vi "Pockels Cal-Reload file.vi"(8 "error in (no error)":errorcluster, 11 "Cal files listbox":refnum<vi>) -> (0 "error out":errorcluster, 3 "All data loaded":string[][](array[string]))   [LabVIEW 2020]
uses:
  Typedefs/Which path.ctl
  <userlib>/My Palettes.lib/Files & paths/Spreadsheet/Read From Spreadsheet File (string)-Mod.vi
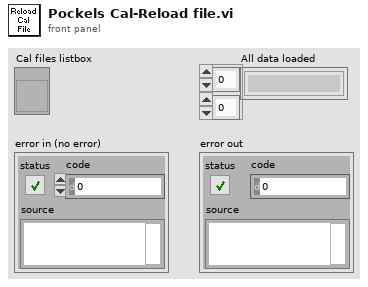
[diagram p1: front panel]
types:
  T1 = typedef "Which path.ctl" = enum16{"Configuration Files", "Calibration Files", "Images", "Setup.ini", "Loaded User profile.ini", "User's-Previous session.ini", "New user profile.ini", "Selected User profile.ini", "User profiles folder", "Power meter scaling.txt", "FOV Cal.ini", "Calibration.ini"}
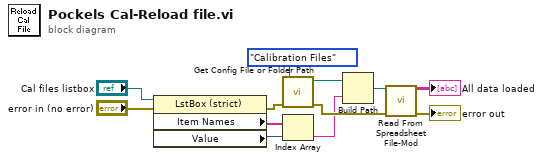
[diagram p0: block diagram]
diagram:
  n1 = property on="Property Node" class="LstBox (strict)"(reference="Cal files listbox", error in="error in (no error)") -> (error out=w10:errorcluster, "Item Names"=w5:string[], "Value"=w6:i32)  [unwired: 1 out]
  n2 = call "Get Config File or Folder Path.vi"("Error In"=w10, "Which file or folder?"=Which_path."Calibration Files" ("Which path?")) -> ("Error Out"=w8:errorcluster, "File Path"=w2:path)  [unwired: 7 in, 1 out]
  n3 = Index Array(array=w5, index=w6) -> (element=w4:string)
  n4 = Build Path(base path=w2, name or relative path=w4) -> (appended path=w3:path)
  n5 = call-poly <userlib>:"Read From Spreadsheet File-Mod.vi"("file path (dialog if empty)"=w3, "error in"=w8) -> ("all rows"=→"All data loaded":string[][], "error out"=→"error out":errorcluster)  [unwired: 8 in, 4 out]
